vi "DSF.Engine.Plugin.Thread.vi"(8 "error in (no error)":errorcluster, 10 "Thread Parameters":refnum<class "Thread Parameters.lvclass">, 11 "Plugin in":refnum<class "DSF.Engine.Plugin.lvclass">) -> (0 "error out":errorcluster, 3 "Plugin out":refnum<class "DSF.Engine.Plugin.lvclass">)   [LabVIEW 2017, in "DSF.Engine.lvlib" / "DSF.Engine.Plugin.lvclass"]
uses:
  DSF.Engine.Plugin.lvclass
  Thread Parameters/Thread Parameters.lvclass
  Thread Parameters/Thread Parameters.lvclass/Thread Parameters.ctl
  <vilib>/Platform/TimedLoop/XDataNode/timing_clust.ctl
  <vilib>/Platform/TimedLoop/XDataNode/nitl_modes.ctl
  <vilib>/Platform/TimedLoop/XDataNode/wakeup.ctl
  <vilib>/platform/TimedLoop/XDataNode/XDataNode.xnode
  <vilib>/Platform/TimedLoop/XDataNode/XDNodeRunTimeDep.lvlib
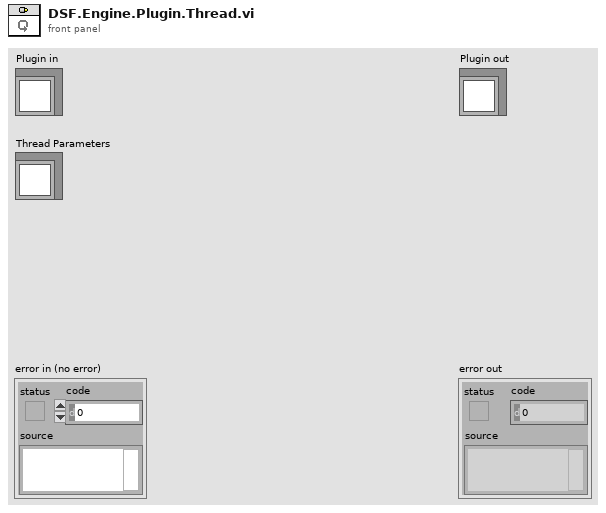
[diagram p1: front panel]
types:
  T1 = typedef "XDNodeRunTimeDep.lvlib/timing_clust.ctl" = cluster{"Expected End [f-1]":u64, "Actual End [f-1]":u64, "Finished Late? [f-1]":bool, "Expected End [i-1]":u64, "Actual End [i-1]":u64, "Finished Late? [i-1]":bool, "Expected Start [i]":u64, "Actual Start [i]":u64, "Expected Start [f]":u64, "Actual Start [f]":u64, "Source Name":string, "Structure Name":string, "Period":i64, "Deadline":i64, "Offset":i64, "Start":i64, "Priority":i32, "Timeout":i32, "Mode":T2, "Wakeup Reason":T3, "Error":errorcluster, "Source Type":string, "Secondary Source Type":string, "Global End Time":u64, "Global Start Time":u64, "Frame Duration":u64, "Iteration Duration":u64, "Assigned CPU":i32, "I/O Scan Engine Mode":u32}
  T2 = typedef "XDNodeRunTimeDep.lvlib/nitl_modes.ctl" = enum32{"No Change", "Process missed periods, maintain original phase", "Discard missed periods, maintain original phase", "Process missed periods, ignore original phase", "Discard missed periods, ignore original phase"}
  T3 = typedef "XDNodeRunTimeDep.lvlib/wakeup.ctl" = enum32{"Normal", "Aborted", "Asynchronous wakeup", "Timing source error", "Timed loop error", "Timeout"}
  T4 = typedef "DSF.Engine.lvlib/DSF.Engine.Interface.Plugin.lvclass/DSF.Engine.Interface.Plugin.Command Data.ctl" = cluster{"Command":T5, "Command Parameters":T6}
  T5 = typedef "DSF.Engine.lvlib/DSF.Engine.Interface.Plugin.lvclass/DSF.Engine.Interface.Plugin.Command.ctl" = enum8{"Rx", "Tx", "Shutdown"}
  T6 = typedef "DSF.Engine.lvlib/DSF.Engine.Interface.Plugin.lvclass/DSF.Engine.Interface.Plugin.Command Parameters.ctl" = cluster{"arg1":u64, "arg2":u64}
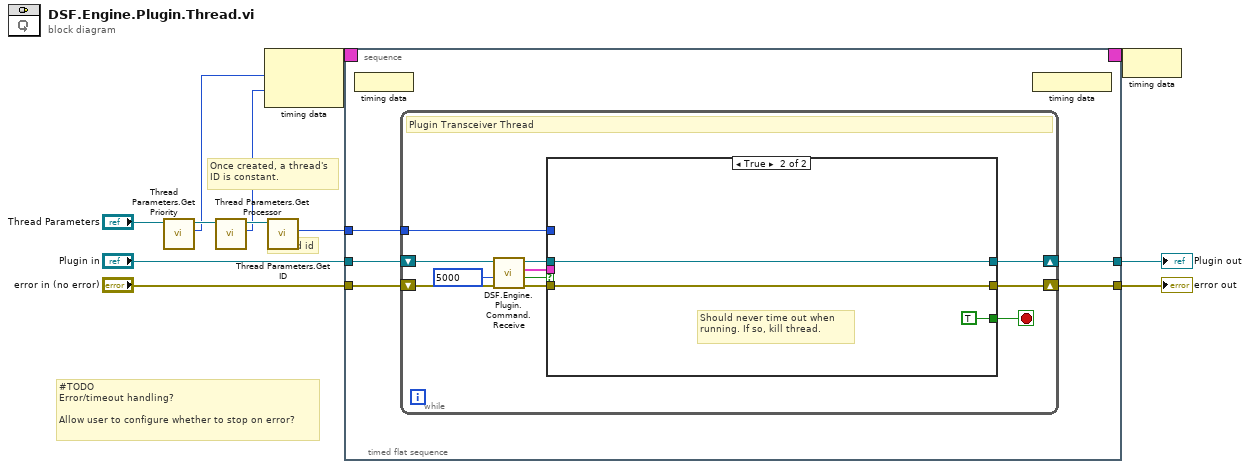
[diagram p0: block diagram]
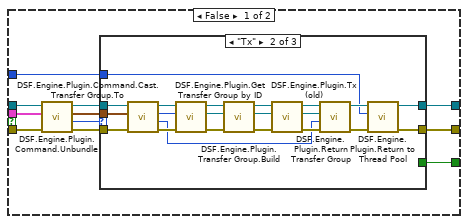
[diagram p2: hidden frame]
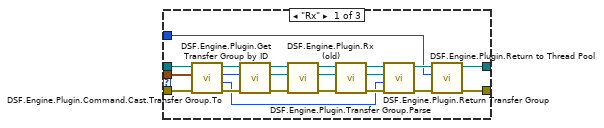
[diagram p3: hidden frame]
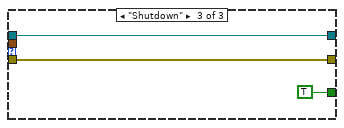
[diagram p4: hidden frame]
diagram:
  # "Once created, a thread's ID is constant."
  # "thread id"
  # "#TODO\nError/timeout handling?\n\nAllow user to configure whether to stop on error?"
  n1 = call "Thread Parameters.Get Priority.vi"("Thread Parameters in"="Thread Parameters") -> ("Priority"=w8:i32, "Thread Parameters out"=w11:refnum<class "Thread Parameters.lvclass">)  [unwired: 9 in]
  n2 = call "Thread Parameters.Get Processor.vi"("Thread Parameters in"=w11) -> ("Processor"=w2:i32, "Thread Parameters out"=w3:refnum<class "Thread Parameters.lvclass">)  [unwired: 9 in]
  n3 = node-c288(w8, w2) -> (w10:T1)
  n4 = call "Thread Parameters.Get ID.vi"("Plugin in"=w3) -> ("id"=w1:i32)  [unwired: 9 in, 1 out]
  n5 = timed-sequence {
    timing: w10 -> [_]
    timing-out: [_] -> w9
    tunnel: "Plugin in" -> [w17]
    tunnel: [w16] -> w6
    tunnel: "error in (no error)" -> [w15]
    tunnel: [w14] -> w4
    tunnel: w1 -> [w13]
    n6 = timed-flat-sequence {
      tunnel: w17 -> [w22]
      tunnel: [w21] -> w16
      tunnel: w15 -> [w20]
      tunnel: [w19] -> w14
      tunnel: w13 -> [w18]
      n7 = node-c288() -> ()  [unwired: 1 in]
      n8 = while {
        shift-right: [w26] -> w19
        shift-left: w20 -> [w29]
        tunnel: w18 -> [w24]
        shift-right: [w30] -> w21
        shift-left: w22 -> [w33]
        stop <- w25 stop-if-true
        # "Plugin Transceiver Thread"
        n9 = call "DSF.Engine.Plugin.Command.Receive.vi"("error in (no error)"=w29, "timeout in ms (0)"=5000 ("timeout in ms"), "Plugin in"=w33) -> ("error out"=w28:errorcluster, "timed out?"=w23:bool, "command"=w27:T4, "Plugin out"=w31:refnum<class "DSF.Engine.Plugin.lvclass">)  [unwired: 5 in]
        n10 = case shown="True" w23 {
          tunnel: w31 -> [w40 w91]
          tunnel: [w44 w91] -> w30
          tunnel: w28 -> [w39 w90]
          tunnel: w27 -> [w38 _]
          tunnel: [w43 w90] -> w26
          tunnel: [w42 TRUE] -> w25
          tunnel: w24 -> [w41 _]
          frame False {
            n11 = call "DSF.Engine.Plugin.Command.Unbundle.vi"("error in (no error)"=w39, "command"=w38, "Plugin in"=w40) -> ("error out"=w36:errorcluster, "command"=w37:T5, "command parameters"=w34:T6, "Plugin out"=w35:refnum<class "DSF.Engine.Plugin.lvclass">)  [unwired: 5 in]
            n12 = case shown="\"Tx\"" w37 {
              tunnel: w35 -> [w65 w86 w89]
              tunnel: [w48 w70 w89] -> w44
              tunnel: w36 -> [w63 w85 w88]
              tunnel: w34 -> [w64 w76 _]
              tunnel: [w47 w69 w88] -> w43
              tunnel: [_ _ TRUE] -> w42
              tunnel: w41 -> [w45 w68 _]
              frame "Rx" {
                n13 = call "DSF.Engine.Plugin.Command.Cast.Transfer Group.To.vi"("error in (no error)"=w63, "command parameters"=w64, "Plugin in"=w65) -> ("error out"=w60:errorcluster, "Transfer Group iteration"=w46:u64, "Transfer Group id"=w61:i32, "Plugin out"=w62:refnum<class "DSF.Engine.Plugin.lvclass">)  [unwired: 5 in]
                n14 = call "DSF.Engine.Plugin.Get Transfer Group by ID.vi"("error in (no error)"=w60, "Transfer Group id"=w61, "Plugin in"=w62) -> ("error out"=w58:errorcluster, "Transfer Group"=w57:refnum<class "DSF.Engine.Transfer Group.lvclass">, "Plugin out"=w59:refnum<class "DSF.Engine.Plugin.lvclass">)  [unwired: 6 in]
                n15 = call "DSF.Engine.Plugin.Rx (old).vi"("error in (no error)"=w58, "Transfer Group in"=w57, "Plugin in"=w59) -> ("error out"=w55:errorcluster, "Transfer Group out"=w54:refnum<class "DSF.Engine.Transfer Group.lvclass">, "Plugin out"=w56:refnum<class "DSF.Engine.Plugin.lvclass">)  [unwired: 6 in]
                n16 = call "DSF.Engine.Plugin.Transfer Group.Parse.vi"("error in (no error)"=w55, "Transfer Group in"=w54, "Plugin in"=w56) -> ("error out"=w52:errorcluster, "Transfer Group out"=w51:refnum<class "DSF.Engine.Transfer Group.lvclass">, "Plugin out"=w53:refnum<class "DSF.Engine.Plugin.lvclass">)  [unwired: 6 in]
                n17 = call "DSF.Engine.Plugin.Return Transfer Group.vi"("error in (no error)"=w52, "Transfer Group iteration"=w46, "Transfer Group"=w51, "Plugin in"=w53) -> ("error out"=w49:errorcluster, "Plugin out"=w50:refnum<class "DSF.Engine.Plugin.lvclass">)  [unwired: 6 in]
                n18 = call "DSF.Engine.Plugin.Return to Thread Pool.vi"("error in (no error)"=w49, "thread id"=w45, "Plugin in"=w50) -> ("error out"=w47:errorcluster, "Plugin out"=w48:refnum<class "DSF.Engine.Plugin.lvclass">)  [unwired: 7 in]
              }
              frame "Tx" {
                n19 = call "DSF.Engine.Plugin.Command.Cast.Transfer Group.To.vi"("error in (no error)"=w85, "command parameters"=w76, "Plugin in"=w86) -> ("error out"=w82:errorcluster, "Transfer Group iteration"=w67:u64, "Transfer Group id"=w83:i32, "Plugin out"=w84:refnum<class "DSF.Engine.Plugin.lvclass">)  [unwired: 5 in]
                n20 = call "DSF.Engine.Plugin.Get Transfer Group by ID.vi"("error in (no error)"=w82, "Transfer Group id"=w83, "Plugin in"=w84) -> ("error out"=w77:errorcluster, "Transfer Group"=w80:refnum<class "DSF.Engine.Transfer Group.lvclass">, "Plugin out"=w81:refnum<class "DSF.Engine.Plugin.lvclass">)  [unwired: 6 in]
                n21 = call "DSF.Engine.Plugin.Transfer Group.Build.vi"("error in (no error)"=w77, "Transfer Group in"=w80, "Plugin in"=w81) -> ("error out"=w78:errorcluster, "Transfer Group out"=w66:refnum<class "DSF.Engine.Transfer Group.lvclass">, "Plugin out"=w79:refnum<class "DSF.Engine.Plugin.lvclass">)  [unwired: 6 in]
                n22 = call "DSF.Engine.Plugin.Tx (old).vi"("error in (no error)"=w78, "Transfer Group in"=w66, "Plugin in"=w79) -> ("error out"=w74:errorcluster, "Transfer Group out"=w73:refnum<class "DSF.Engine.Transfer Group.lvclass">, "Plugin out"=w75:refnum<class "DSF.Engine.Plugin.lvclass">)  [unwired: 6 in]
                n23 = call "DSF.Engine.Plugin.Return Transfer Group.vi"("error in (no error)"=w74, "Transfer Group iteration"=w67, "Transfer Group"=w73, "Plugin in"=w75) -> ("error out"=w71:errorcluster, "Plugin out"=w72:refnum<class "DSF.Engine.Plugin.lvclass">)  [unwired: 6 in]
                n24 = call "DSF.Engine.Plugin.Return to Thread Pool.vi"("error in (no error)"=w71, "thread id"=w68, "Plugin in"=w72) -> ("error out"=w69:errorcluster, "Plugin out"=w70:refnum<class "DSF.Engine.Plugin.lvclass">)  [unwired: 7 in]
              }
              frame "Shutdown" {
              }
            }
          }
          frame True {
            # "Should never time out when running. If so, kill thread."
          }
        }
      }
      n25 = node-c288() -> ()  [unwired: 1 out]
    }
  }
  "error out" <- w4
  "Plugin out" <- w6
  n26 = node-c288(w9) -> ()
